vi "Stop Core.vi"(10 "final error code":i32, 11 "Arduino_Stepper in":refnum<class "Arduino_Stepper.lvclass">) -> (3 "Arduino_Stepper out":refnum<class "Arduino_Stepper.lvclass">)   [LabVIEW 2023, in "Arduino_TranslationStage_UI.lvlib" / "Arduino_Stepper.lvclass"]
doc: "(<B>Filename</B>: Actor Framework.lvlib:Actor.lvclass:Stop Core.vi)\n\nDefines what the actor does before it stops. Use the <B>final error code</B> input to determine whether the actor shut down in response to an error.\n\nBy default, this method passes the Stop message along to all auto-stop nested actors. A descendant class may override this method to define additional behavior, such as shutting down any processes the actor initiated in its override of the Actor Core method."
uses:
  Arduino_Stepper.lvclass
  Arduino_Stepper.lvclass/Arduino_Stepper.ctl
  <vilib>/ActorFramework/Actor/Actor.lvclass
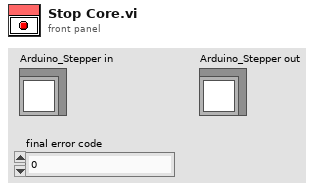
[diagram p1: front panel]
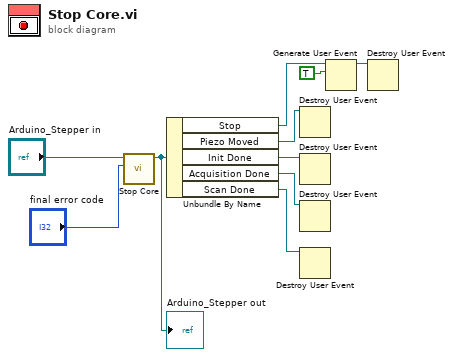
[diagram p0: block diagram]
diagram:
  n1 = call-parent "Stop Core.vi"("final error code"="final error code", "Actor in"="Arduino_Stepper in") -> ("Actor out"=w1:refnum<class "Arduino_Stepper.lvclass">)  [unwired: 9 in]
  "Arduino_Stepper out" <- w1
  n2 = Unbundle By Name(w1) -> ("Stop"=w8:refnum<user-event>, "Piezo Moved"=w5:refnum<user-event>, "Init Done"=w4:refnum<user-event>, "Acquisition Done"=w2:refnum<user-event>, "Scan Done"=w3:refnum<user-event>)
  n3 = Destroy User Event(user event=w5) -> ()  [unwired: 1 in, 1 out]
  n4 = Destroy User Event(user event=w4) -> ()  [unwired: 1 in, 1 out]
  n5 = Destroy User Event(user event=w2) -> ()  [unwired: 1 in, 1 out]
  n6 = Destroy User Event(user event=w3) -> ()  [unwired: 1 in, 1 out]
  n7 = Generate User Event(user event=w8, event data cluster=TRUE ("event data")) -> (user event out=w6:refnum<user-event>)  [unwired: 2 in, 1 out]
  n8 = Destroy User Event(user event=w6) -> ()  [unwired: 1 in, 1 out]
